vi "Periodic Tasks.vi"(8 "error in":errorcluster) -> ()   [LabVIEW 2019]
doc: "This VI runs in parallel to other robot code. It can contain as many user-defined periodic loops as you need. These can carry out PID or other sorts of timed response."
uses:
  <vilib>/Rock Robotics/WPI/Utilities/WPI_GetSetVariantRefNum.vi
  Robot Global Data.vi
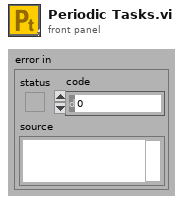
[diagram p1: front panel]
types:
  T1 = typedef "WPI_JoystickDevRef.ctl" = cluster{"Device":T2}
  T2 = typedef "WPI_JoystickDeviceEnum.ctl" = enum16{"USB 0", "USB 1", "USB 2", "USB 3", "USB 4", "USB 5"}
  T3 = cluster{"JoystickDevRef":T1, "JoystickDevRef":T1}
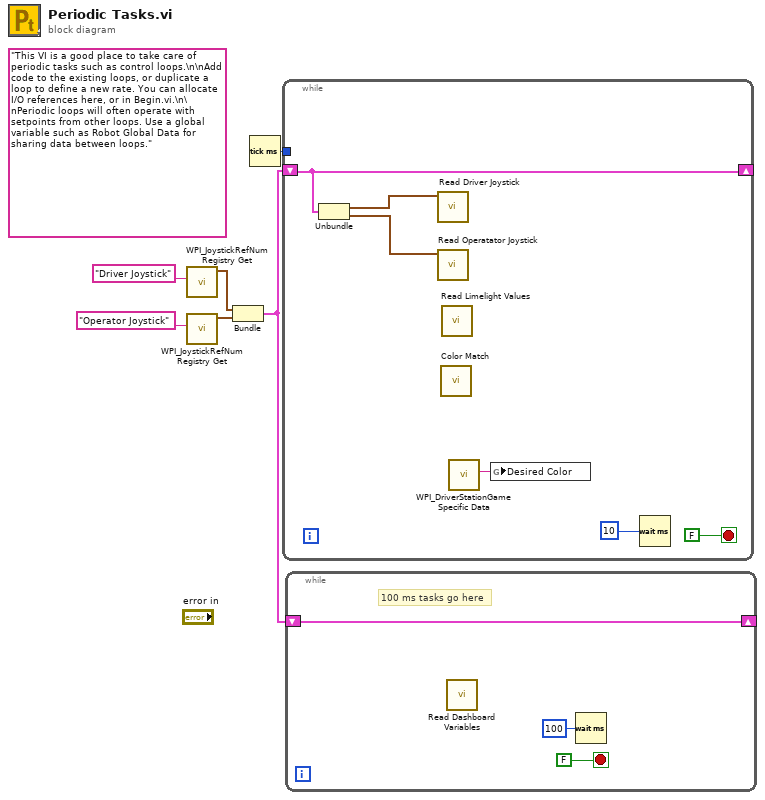
[diagram p0: block diagram]
diagram:
  (unwired) "This VI is a good place to take care of periodic tasks such as control loops.\n\nAdd code to the existing loops, or duplicate a loop to define a new rate. You can allocate I/O references here, or in Begin.vi.\n\nPeriodic loops will often operate with setpoints from other loops. Use a global variable such as Robot Global Data for sharing data between loops."
  n1 = call <vilib>:"WPI_JoystickRefNum Registry Get.vi"("refnum name"="Driver Joystick") -> ("JoystickDevRef"=w2:T1)  [unwired: 1 in, 9 out]
  n2 = call <vilib>:"WPI_JoystickRefNum Registry Get.vi"("refnum name"="Operator Joystick") -> ("JoystickDevRef"=w3:T1)  [unwired: 1 in, 9 out]
  n3 = Bundle("JoystickDevRef"=w2, "JoystickDevRef"=w3) -> (w1:T3)  [unwired: 1 in]
  n4 = Tick Count (ms)() -> (millisecond timer value=w5:u32)
  n5 = while {
    shift-right: [w10] -> _
    shift-left: w1 -> [w10]
    tunnel: w5 -> [_]
    stop <- FALSE stop-if-true
    n6 = Unbundle(w10) -> ("JoystickDevRef"=w9:T1, "JoystickDevRef"=w8:T1)
    n7 = call "Read Driver Joystick.vi"("Driver Joystick"=w9) -> ()  [unwired: 11 in]
    n8 = call "Read Operatator Joystick.vi"("Operator Joystick"=w8) -> ()  [unwired: 11 in]
    n9 = call "Color Match.vi"() -> ()  [unwired: 12 in]
    n10 = call "Read Limelight Values.vi"() -> ()  [unwired: 12 in]
    n11 = call <vilib>:"WPI_DriverStationGame Specific Data.vi"() -> ("Game Specific Data"=w7:string)  [unwired: 11 in]
    n12 = global write "Robot Global Data.vi" "Desired Color"(w7) -> ()
    n13 = Wait (ms)(milliseconds to wait=u32 10) -> ()  [unwired: 1 out]
  }
  n14 = while {
    shift-right: [w13] -> _
    shift-left: w1 -> [w13]
    stop <- FALSE stop-if-true
    # "100 ms tasks go here"
    n15 = call "Read Dashboard Variables.vi"() -> ()  [unwired: 12 in]
    n16 = Wait (ms)(milliseconds to wait=u32 100) -> ()  [unwired: 1 out]
  }
